vi "AI Config Pane.vi"(6 "_SubPanelMessages":refnum<notifier>, 9 "_myEmbeddedToFrameEvent":T7, 10 "_myEmbedded.Exit":refnum<user-event>, 11 "-Property Bundle":cluster{"Name":string, "Value":variant}[](array[cluster])) -> (1 "_Connection Informations":T1, 2 "_Scripter Input":T9)   [LabVIEW 2021]
uses:
  <vilib>/myRIO/Common/Express VI Framework/xctls/myRIO Channel List/myRIO Channel List.xctl
  <vilib>/myRIO/Common/Express VI Framework/typedefs/Config Pane to Framework Ref.ctl
  <vilib>/myRIO/Common/Express VI Framework/typedefs/Data Validate Ref.ctl
  <vilib>/myRIO/Common/Express VI Framework/typedefs/Scripter Input.ctl
  <vilib>/myRIO/Common/Express VI Framework/typedefs/WireThrough Terminal Names.ctl
  <vilib>/myRIO/Common/Express VI Framework/typedefs/Instrument Driver Method Descriptor Array.ctl
  <vilib>/myRIO/Common/Express VI Framework/typedefs/Instrument Driver Method Descriptor.ctl
  <vilib>/myRIO/Common/Express VI Framework/typedefs/Sub Panel Messages.ctl
  <vilib>/myRIO/Common/Express VI Framework/typedefs/Connection Informations.ctl
  <vilib>/myRIO/Common/Instrument Driver Framework/Utilities/typedefs/Channel Types.ctl
  <vilib>/myRIO/Common/Profile Manager Framework/typedefs/Channel Type Profile.ctl
  <vilib>/myRIO/Common/Profile Manager Framework/typedefs/Channel Info.ctl
panel:
  in  "Range Indexes":i32[](array[numeric])
  in  "Selected Channel List":T2[](xcontrol)=[{"Channel Name"=0, "Channel Alias"="", "Remove Channel"=FALSE, "Index"=0}]
  in  "_Default Alias String":string
  in  "_VI Default Name (Edit and make value default)":string="Analog input (1 sample)"
  in  "Name:":string caption="Node name:"
  in  "_WireThrough Info (Edit and make value default)":T4={"WireThrough Top In"="AI Ref In", "WireThrough Bottom In"="error in (no error)", "WireThrough Top Out"="AI Ref Out", "WireThrough Bottom Out"="error out"}
  in  "_Template Array (Edit and make value default)":T5=[{"Function Name"="Smart Open", "VI Path"=path "<vilib>/myRIO/Instrument Drivers/Onboard IO/AI/vis", "Script"=TRUE, "Inputs"=[{"name"="Channel Names", "value"=variant, "Config Pane Only"=TRUE, "Build Array"=FALSE, "Bundle Cluster"=FALSE, "Show Term"=FALSE, "alias"=[], "Required Input"=FALSE}], "Outputs"=[], "VI Class"=enum."Open", "Controls Refs[]"=[], "Inline"=FALSE}, {"Function Name"="Open", "VI Path"=path "<vilib>/myRIO/Instrument Drivers/Onboard IO/AI/vis", "Script"=FALSE, "Inputs"=[{"name"="Channel Names", "value"=variant, "Config Pane Only"=TRUE, "Build Array"=FALSE, "Bundle Cluster"=FALSE, "Show Term"=FALSE, "alias"=[], "Required Input"=FALSE}], "Outputs"=[], "VI Class"=enum."Open", "Controls Refs[]"=[], "Inline"=FALSE}, {"Function Name"="Read", "VI Path"=path "<vilib>/myRIO/Instrument Drivers/Onboard IO/AI/vis", "Script"=TRUE, "Inputs"=[], "Outputs"=[{"name"="Values", "value"=variant, "Show Term"=TRUE, "Index Array"=TRUE, "Unbundle Cluster"=FALSE, "alias"=[]}], "VI Class"=enum."Data", "Controls Refs[]"=[], "Inline"=FALSE}, {"Function Name"="Close", "VI Path"=path "<vilib>/myRIO/Instrument Drivers/Onboard IO/AI/vis", "Script"=FALSE, "Inputs"=[], "Outputs"=[], "VI Class"=enum."Close", "Controls Refs[]"=[], "Inline"=FALSE}]
  in  "_Test Close":bool
  # "User Visible Area"
  # "NOTE: Tab Order has been set\nfor this Front Panel.\n1. Name: (string control)\n2. Add Channel (button)\n3. Selected Channel List (array)\n\nAll other controls are excluded \nfrom Tabbing order\n\nTo exlude a control from context\nhelp prefix its label text with a '-'"
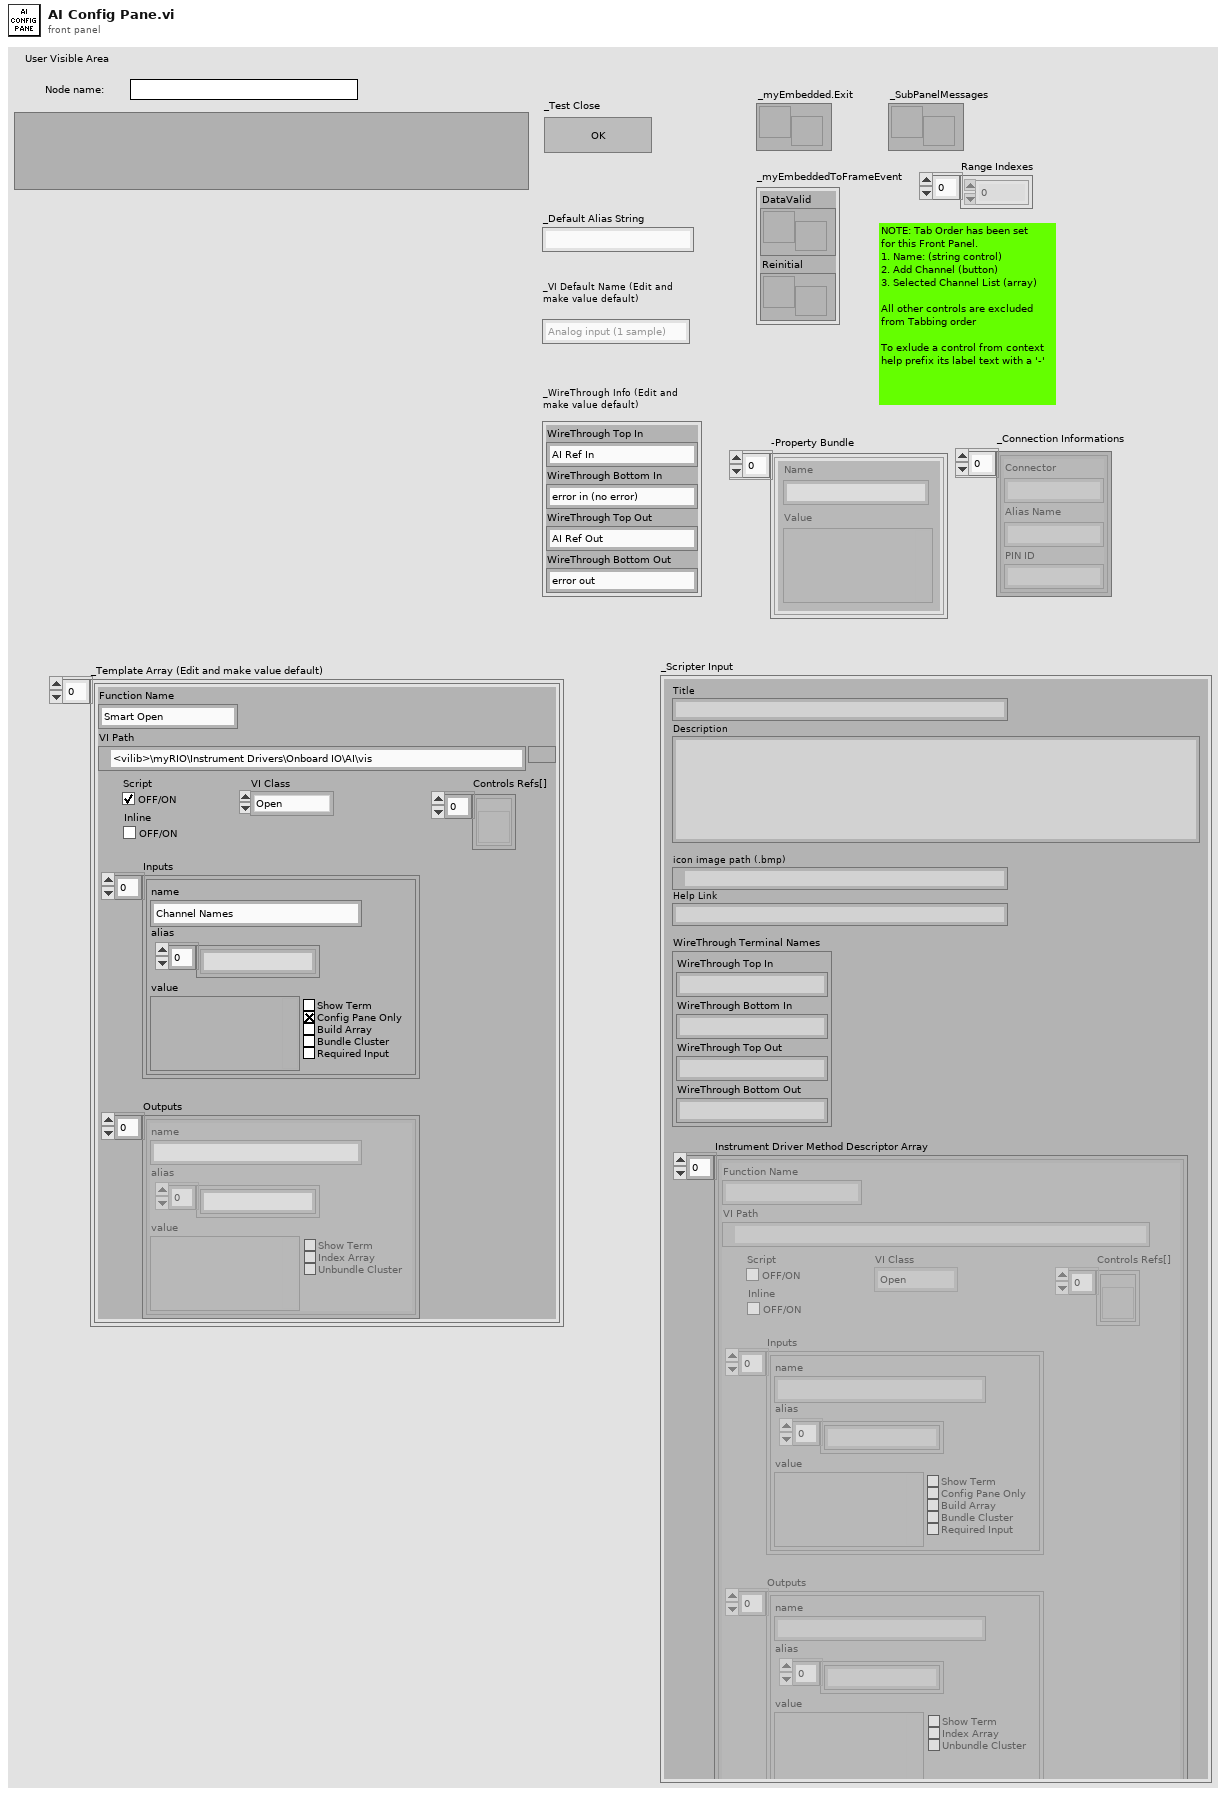
[diagram p1: front panel]
types:
  T1 = typedef "Connection Informations.ctl" = cluster{"Connector":string, "Alias Name":string, "PIN ID":string}[]
  T2 = typedef "myRIO Channel List.xctl/Channel Data.ctl" = cluster{"Channel Name":u16, "Channel Alias":string, "Remove Channel":T3, "Index":i32}
  T3 = typedef "myRIO Channel List.xctl/Remove Channel.ctl" = bool
  T4 = typedef "WireThrough Terminal Names.ctl" = cluster{"WireThrough Top In":string, "WireThrough Bottom In":string, "WireThrough Top Out":string, "WireThrough Bottom Out":string}
  T5 = typedef "Instrument Driver Method Descriptor Array.ctl" = T6[]
  T6 = typedef "Instrument Driver Method Descriptor.ctl" = cluster{"Function Name":string, "VI Path":path, "Script":bool, "Inputs":cluster{"name":string, "value":variant, "Config Pane Only":bool, "Build Array":bool, "Bundle Cluster":bool, "Show Term":bool, "alias":string[], "Required Input":bool}[], "Outputs":cluster{"name":string, "value":variant, "Show Term":bool, "Index Array":bool, "Unbundle Cluster":bool, "alias":string[]}[], "VI Class":enum16{"Open", "Configure", "Data", "Manage", "Close"}, "Controls Refs[]":refnum<vi>[], "Inline":bool}
  T7 = typedef "Config Pane to Framework Ref.ctl" = cluster{"DataValid":T8, "Reinitial":refnum<user-event>}
  T8 = typedef "Data Validate Ref.ctl" = refnum<user-event>
  T9 = typedef "Scripter Input.ctl" = cluster{"Title":string, "Description":string, "icon image path (.bmp)":path, "Help Link":string, "WireThrough Terminal Names":T4, "Instrument Driver Method Descriptor Array":T5}
  T10 = typedef "Channel Types.ctl" = enum32{"Unknown", "AI", "AO", "DIO - DI", "DIO", "DIO - DO", "I2C", "PWM", "Encoder", "SPI", "UART", "Accelerometer", "DIO - LED", "DIO - Button", "AI (N Samples)", "AudioIn (N Samples)", "AO (N Samples)", "AudioOut (N Samples)", "DI (N Samples)", "DO (N Samples)", "AI IRQ", "DI IRQ", "Timer IRQ", "RSL", "Relay", "CAN", "AI (Continuous)", "AO (Continuous)"}
  T11 = typedef "Channel Type Profile.ctl" = cluster{"Channel Type":T10, "No. of Channels":dbl, "Channel List":T12[]}
  T12 = typedef "Channel Info.ctl" = cluster{"Channel Name":string, "Alias":string, "Used?":bool, "Not Support?":bool, "Property Bundle":cluster{"Name":string, "Value":variant}[]}
  T13 = typedef "Sub Panel Messages.ctl" = enum16{"Initialized"}
  T14 = cluster{"name":string, "value":variant, "Config Pane Only":bool, "Build Array":bool, "Bundle Cluster":bool, "Show Term":bool, "alias":string[], "Required Input":bool}
  T15 = cluster{"Connector":string, "Alias Name":string, "PIN ID":string}[]
  T16 = cluster{"name":string, "value":variant, "Config Pane Only":bool, "Build Array":bool, "Bundle Cluster":bool, "Show Term":bool, "alias":string[], "Required Input":bool}[]
  T17 = cluster{"name":string, "value":variant, "Show Term":bool, "Index Array":bool, "Unbundle Cluster":bool, "alias":string[]}[]
  T18 = cluster{"name":string, "value":variant, "Show Term":bool, "Index Array":bool, "Unbundle Cluster":bool, "alias":string[]}
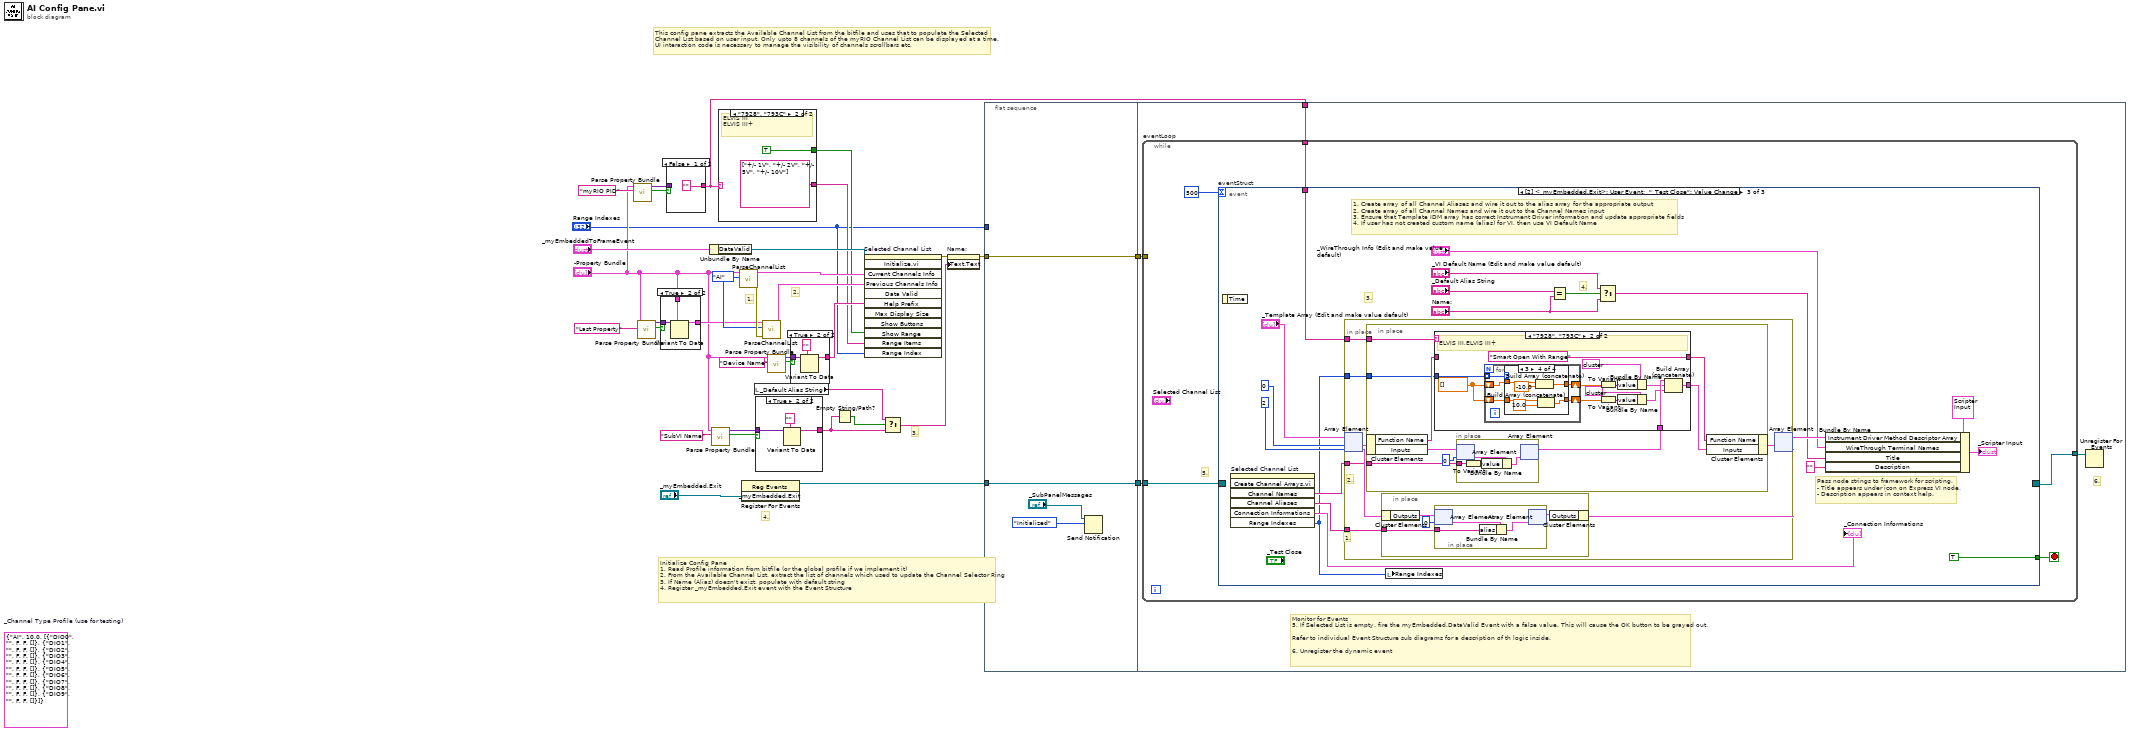
[diagram p0: block diagram]
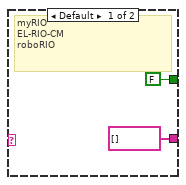
[diagram p2: hidden frame]
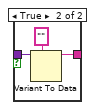
[diagram p3: hidden frame]
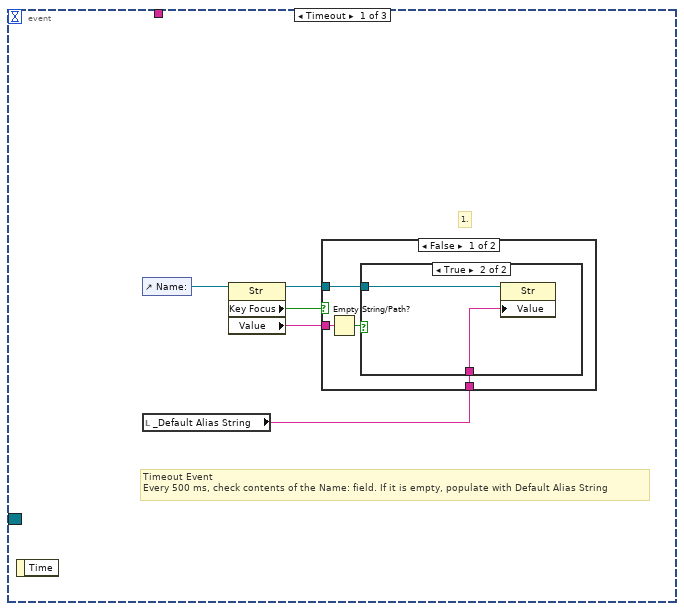
[diagram p4: hidden frame]
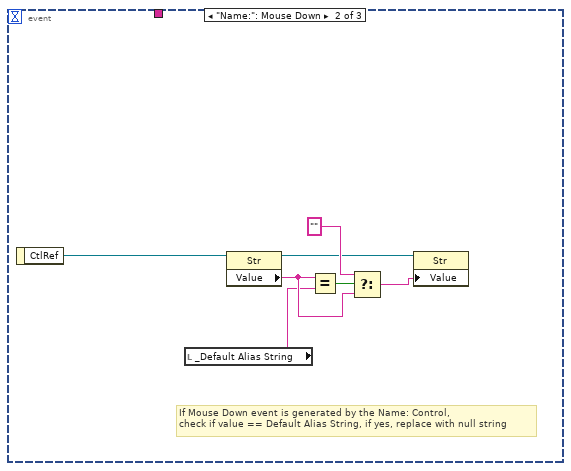
[diagram p7: hidden frame]
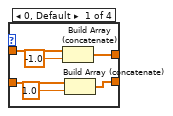
[diagram p9: hidden frame]
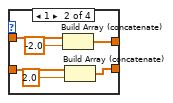
[diagram p10: hidden frame]
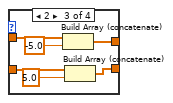
[diagram p11: hidden frame]
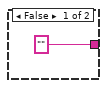
[diagram p14: hidden frame]
diagram:
  w18 = Channel_Types."AI" ("Channel to Read")
  (unwired) T11 {"Channel Type"=enum."AI", "No. of Channels"=10.0, "Channel List"=[{"Channel Name"="DIO0", "Alias"="", "Used?"=FALSE, "Not Support?"=FALSE, "Property Bundle"=[]}, {"Channel Name"="DIO1", "Alias"="", "Used?"=FALSE, "Not Support?"=FALSE, "Property Bundle"=[]}, {"Channel Name"="DIO2", "Alias"="", "Used?"=FALSE, "Not Support?"=FALSE, "Property Bundle"=[]}, {"Channel Name"="DIO3", "Alias"="", "Used?"=FALSE, "Not Support?"=FALSE, "Property Bundle"=[]}, {"Channel Name"="DIO4", "Alias"="", "Used?"=FALSE, "Not Support?"=FALSE, "Property Bundle"=[]}, {"Channel Name"="DIO5", "Alias"="", "Used?"=FALSE, "Not Support?"=FALSE, "Property Bundle"=[]}, {"Channel Name"="DIO6", "Alias"="", "Used?"=FALSE, "Not Support?"=FALSE, "Property Bundle"=[]}, {"Channel Name"="DIO7", "Alias"="", "Used?"=FALSE, "Not Support?"=FALSE, "Property Bundle"=[]}, {"Channel Name"="DIO8", "Alias"="", "Used?"=FALSE, "Not Support?"=FALSE, "Property Bundle"=[]}, {"Channel Name"="DIO9", "Alias"="", "Used?"=FALSE, "Not Support?"=FALSE, "Property Bundle"=[]}]}  # _Channel Type Profile (use for testing)
  # "3."
  # "2."
  # "1."
  # "This config pane extracts the Available Channel List from the bitfile and uses that to populate the Selected \nChannel List based on user input. Only upto 8 channels of the myRIO Channel List can be displayed at a time. \nUI interaction code is necessary to manage the visibility of channels scrollbars etc."
  # "4."
  # "Initialize Config Pane\n1. Read Profile information from bitfile (or the global profile if we implement it)\n2. From the Available Channel List, extract the list of channels which used to update the Channel Selector Ring\n3. If Name (Alias) doesn't exist, populate with default string\n4. Register _myEmbedded.Exit event with the Event Structure"
  n1 = call <vilib>:"Parse Property Bundle.vi"("Name"="myRIO PID", "Property Bundle"="-Property Bundle") -> ("Found?"=w1:bool, "Value"=w7:variant)  [unwired: 8 in]
  n2 = call <vilib>:"Parse Property Bundle.vi"("Name"="Last Property", "Property Bundle"="-Property Bundle") -> ("Found?"=w20:bool, "Value"=w21:variant)  [unwired: 8 in]
  n3 = case shown="True" w20 {
    tunnel: w21 -> [_ w38]
    tunnel: [_ w37] -> w17
    tunnel: "-Property Bundle" -> [_ w36]
    frame False {
    }
    frame True {
      n4 = Variant To Data(type=w36, Variant=w38) -> (data=w37:cluster{"Name":string, "Value":variant}[])  [unwired: 1 in, 1 out]
    }
  }
  n5 = case shown="False" w1 {
    tunnel: w7 -> [_ w42]
    tunnel: ["" ("Name") w41] -> w2
    frame False {
    }
    frame True {
      n6 = Variant To Data(type="" ("Name"), Variant=w42) -> (data=w41:string)  [unwired: 1 in, 1 out]
    }
  }
  n7 = Unbundle By Name("_myEmbeddedToFrameEvent") -> ("DataValid"=w11:T8)
  n8 = call <vilib>:"Parse Property Bundle.vi"("Name"="SubVI Name", "Property Bundle"="-Property Bundle") -> ("Found?"=w29:bool, "Value"=w30:variant)  [unwired: 8 in]
  n9 = case shown="\"7928\", \"793C\"" w2 {
    tunnel: [FALSE TRUE] -> w4
    tunnel: [string[] [] ("Range Items") string[] ["+/- 1V", "+/- 2V", "+/- 5V", "+/- 10V"] ("Range Items")] -> w5
    frame Default {
      # "myRIO\nEL-RIO-CM\nroboRIO"
    }
    frame "7928", "793C" {
      # "ELVIS III\nELVIS III+"
    }
  }
  n10 = call <vilib>:"ParseChannelList.vi"("Channel to Read"=w18, "_Property Bundle"="-Property Bundle") -> ("error out"=w19:errorcluster, "Channel List Out"=w23:T12[])  [unwired: 7 in, 1 out]
  n11 = register-events("_myEmbedded.Exit") -> (reference out=w27:refnum<event-registration>)  [unwired: 2 in, 1 out]
  n12 = local read "_Default Alias String"() -> (w25:string)
  n13 = case shown="True" w29 {
    tunnel: w30 -> [_ w50]
    tunnel: ["" ("Name") w48] -> w28
    frame False {
    }
    frame True {
      n14 = Variant To Data(type="" ("Name"), Variant=w50) -> (data=w48:string)  [unwired: 1 in, 1 out]
    }
  }
  n15 = call <vilib>:"ParseChannelList.vi"("error in (no error)"=w19, "Channel to Read"=w18, "_Property Bundle"=w17) -> ("Channel List Out"=w16:T12[])  [unwired: 6 in, 2 out]
  n16 = call <vilib>:"Parse Property Bundle.vi"("Name"="Device Name", "Property Bundle"="-Property Bundle") -> ("Found?"=w15:bool, "Value"=w14:variant)  [unwired: 8 in]
  n17 = case shown="True" w15 {
    tunnel: w14 -> [_ w53]
    tunnel: [_ w52] -> w12
    frame False {
    }
    frame True {
      n18 = Variant To Data(type="", Variant=w53) -> (data=w52:string)  [unwired: 1 in, 1 out]
    }
  }
  n19 = Empty String/Path?(string/path=w28) -> (empty?=w34:bool)
  n20 = invoke on="Selected Channel List" class="myRIO Channel List (strict)" method="Initialize.vi"("Current Channels Info"=w23, "Previous Channels Info"=w16, "Data Valid"=w11, "Help Prefix"=w12, "Show Range"=w4, "Range Items"=w5, "Range Index"="Range Indexes") -> (error out=w26:errorcluster)  [unwired: 5 in, 11 out]
  n21 = Select(t=w25, s=w34, f=w28) -> (s? t:f=w33:string)
  n22 = property on="Name:" class="Str"(error in=w26, "Text.Text"=w33) -> (error out=w32:errorcluster)  [unwired: 1 in, 1 out]
  n23 = flat-sequence {
    tunnel: w27 -> [w56]
    tunnel: w32 -> [w57]
    tunnel: [w57] -> w10
    tunnel: [w56] -> w9
    tunnel: "Range Indexes" -> [_]
    tunnel: w10 -> [w60]
    tunnel: w9 -> [w59]
    tunnel: w2 -> [w58]
    frame #0 {
      n24 = Send Notification(notification=Sub_Panel_Messages."Initialized", notifier="_SubPanelMessages") -> ()  [unwired: 1 in, 2 out]
    }
    frame #1 {
      # "Monitor for Events\n5. If Selected List is empty, fire the myEmbedded.DataValid Event with a false value. This will cause the OK button to be grayed out.\n\nRefer to individual Event Structure sub diagrams for a description of th logic inside.\n\n6. Unregister the dynamic event"
      # "6."
      n25 = while "eventLoop" {
        tunnel: w59 -> [w65]
        tunnel: [w64] -> w61
        tunnel: w60 -> [_]
        tunnel: w58 -> [w62]
        stop <- w66 stop-if-true
        # "5."
        n26 = event "eventStruct" shown="[2] <_myEmbedded.Exit>: User Event;  \"_Test Close\": Value Change" {
          selector: w65 -> [_ _ _]
          dyn-events: [_ _ _] -> w64
          timeout: 500 -> [_ _ _]
          tunnel: [_ _ TRUE ("_Test Close")] -> w66
          tunnel: w62 -> [_ _ w86]
          event Timeout {
            # "Timeout Event\nEvery 500 ms, check contents of the Name: field. If it is empty, populate with Default Alias String"
            # "1."
            n27 = event-data() -> ()  [unwired: 1 in, 1 out]
            n28 = control-ref of="Name:"() -> (w69:refnum<vi>)
            n29 = local read "_Default Alias String"() -> (w67:string)
            n30 = property on="Property Node" class="Str"(reference=w69) -> (reference out=w68:refnum<vi>, "Key Focus"=w70:bool, "Value"=w71:string)  [unwired: 1 in, 1 out]
            n31 = case shown="False" w70 {
              tunnel: w71 -> [w75 _]
              tunnel: w68 -> [w73 _]
              tunnel: w67 -> [w72 _]
              frame False {
                n32 = Empty String/Path?(string/path=w75) -> (empty?=w74:bool)
                n33 = case shown="True" w74 {
                  tunnel: w73 -> [_ w77]
                  tunnel: w72 -> [_ w76]
                  frame False {
                  }
                  frame True {
                    n34 = property on="Property Node" class="Str"(reference=w77, "Value"=w76) -> ()  [unwired: 1 in, 2 out]
                  }
                }
              }
              frame True {
              }
            }
          }
          event "Name:": Mouse Down {
            # "If Mouse Down event is generated by the Name: Control,\ncheck if value == Default Alias String, if yes, replace with null string"
            n35 = event-data() -> ("CtlRef"=w84:refnum<vi>)  [unwired: 1 in]
            n36 = local read "_Default Alias String"() -> (w78:string)
            n37 = property class="Str"(reference=w84) -> (reference out=w80:refnum<vi>, "Value"=w79:string)  [unwired: 1 in, 1 out]
            n38 = Equal?(x=w79, y=w78) -> (x = y?=w83:bool)
            n39 = Select(t="", s=w83, f=w79) -> (s? t:f=w81:string)
            n40 = property class="Str"(reference=w80, "Value"=w81) -> ()  [unwired: 1 in, 2 out]
          }
          event User Event; "_Test Close": Value Change {
            # "2."
            # "1."
            # "1. Create array of all Channel Aliases and wire it out to the alias array for the appropriate output\n2. Create array of all Channel Names and wire it out to the Channel Names input\n3. Ensure that Template IDM array has correct Instrument Driver information and update appropriate fields\n4. If user has not created custom name (alias) for VI, then use VI Default Name"
            # "4."
            # "3."
            # "Pass node strings to framework for scripting.\n- Title appears under icon on Express VI node.\n- Description appears in context help."
            n41 = event-data() -> ()  [unwired: 1 in, 1 out]
            n42 = invoke on="Selected Channel List" class="myRIO Channel List (strict)" method="Create Channel Arrays.vi"() -> ("Channel Names"=w89:string[], "Channel Aliases"=w88:string[], "Connection Informations"=→"_Connection Informations":T15, "Range Indexes"=w85:i32[])  [unwired: 7 in, 3 out]
            n43 = in-place {
              in-place-border: w89 -> [w107]
              in-place-border: w88 -> [w106]
              in-place-border: w86 -> [w105]
              in-place-border: w85 -> [w104]
              n44 = in-place-array #1("_Template Array (Edit and make value default)", 0, 2) -> (w111:T6, w109:T6)
              n45 = in-place {
                in-place-border: w107 -> [w126]
                in-place-border: w105 -> [w124]
                in-place-border: w104 -> [w120]
                n46 = in-place-cluster #2(w111) -> ("Function Name"=w123:string, "Inputs"=w127:T16)
                n47 = in-place {
                  in-place-border: w126 -> [w172]
                  n48 = in-place-array #3(w127, 0) -> (w175:T14)
                  n49 = To Variant(anything=w172) -> (Variant=w173:variant)
                  n50 = Bundle By Name(cluster=w175, "value"=w173) -> (w174:T14)
                  n51 = in-place-array #3(w174) -> (w121:T16)  [unwired: 1 out]
                }
                n52 = case shown="\"7928\", \"793C\"" w124 {
                  tunnel: w123 -> [w129 _]
                  tunnel: [w129 "Smart Open With Range"] -> w122
                  tunnel: w121 -> [w128 w141]
                  tunnel: w120 -> [_ w140]
                  tunnel: [w128 w130] -> w119
                  frame Default {
                    # "myRIO,EL-RIO-CM,roboRIO"
                  }
                  frame "7928", "793C" {
                    w139 = dbl[] []
                    # "ELVIS III,ELVIS III+"
                    n53 = for {
                      tunnel: w140 -> [w147] mode=indexing
                      shift-right: [w145] -> w137
                      shift-left: w139 -> [w146]
                      shift-right: [w143] -> w134
                      shift-left: w139 -> [w144]
                      n54 = case shown="3" w147 {
                        tunnel: w146 -> [w151 w157 w163 w169]
                        tunnel: [w150 w156 w162 w168] -> w145
                        tunnel: w144 -> [w149 w155 w161 w167]
                        tunnel: [w148 w154 w160 w166] -> w143
                        frame 0, Default {
                          n55 = Build Array (concatenate)(w151, -1.0) -> (w150:dbl[])
                          n56 = Build Array (concatenate)(w149, 1.0) -> (w148:dbl[])
                        }
                        frame 1 {
                          n57 = Build Array (concatenate)(w157, -2.0) -> (w156:dbl[])
                          n58 = Build Array (concatenate)(w155, 2.0) -> (w154:dbl[])
                        }
                        frame 2 {
                          n59 = Build Array (concatenate)(w163, -5.0) -> (w162:dbl[])
                          n60 = Build Array (concatenate)(w161, 5.0) -> (w160:dbl[])
                        }
                        frame 3 {
                          n61 = Build Array (concatenate)(w169, -10.0) -> (w168:dbl[])
                          n62 = Build Array (concatenate)(w167, 10.0) -> (w166:dbl[])
                        }
                      }
                    }
                    n63 = To Variant(anything=w137) -> (Variant=w138:variant)
                    n64 = To Variant(anything=w134) -> (Variant=w135:variant)
                    n65 = Bundle By Name(cluster=T14 {"name"="Min Value", "value"=variant, "Config Pane Only"=TRUE, "Build Array"=FALSE, "Bundle Cluster"=FALSE, "Show Term"=FALSE, "alias"=[], "Required Input"=FALSE} ("element"), "value"=w138) -> (w132:T14)
                    n66 = Bundle By Name(cluster=T14 {"name"="Max Value", "value"=variant, "Config Pane Only"=TRUE, "Build Array"=FALSE, "Bundle Cluster"=FALSE, "Show Term"=FALSE, "alias"=[], "Required Input"=FALSE} ("element"), "value"=w135) -> (w131:T14)
                    n67 = Build Array (concatenate)(w141, w132, w131) -> (w130:T16)
                  }
                }
                n68 = in-place-cluster #2("Function Name"=w122, "Inputs"=w119) -> (w110:T6)
              }
              n69 = in-place {
                in-place-border: w106 -> [w114]
                n70 = in-place-cluster #4(w109) -> ("Outputs"=w115:T17)
                n71 = in-place {
                  in-place-border: w114 -> [w116]
                  n72 = in-place-array #5(w115, 0) -> (w118:T18)
                  n73 = Bundle By Name(cluster=w118, "alias"=w116) -> (w117:T18)
                  n74 = in-place-array #5(w117) -> (w113:T17)  [unwired: 1 out]
                }
                n75 = in-place-cluster #4("Outputs"=w113) -> (w108:T6)
              }
              n76 = in-place-array #1(w110, w108) -> (w101:T5)  [unwired: 2 out]
            }
            n77 = local write "Range Indexes"(w85) -> ()
            n78 = Equal?(x="_Default Alias String", y="Name:") -> (x = y?=w93:bool)
            n79 = Select(t="_VI Default Name (Edit and make value default)", s=w93, f="Name:") -> (s? t:f=w91:string)
            n80 = Bundle By Name(cluster=T9 {"Title"="", "Description"="", "icon image path (.bmp)"=path "", "Help Link"="", "WireThrough Terminal Names"={"WireThrough Top In"="", "WireThrough Bottom In"="", "WireThrough Top Out"="", "WireThrough Bottom Out"=""}, "Instrument Driver Method Descriptor Array"=[]} ("Scripter Input"), "Instrument Driver Method Descriptor Array"=w101, "WireThrough Terminal Names"="_WireThrough Info (Edit and make value default)", "Title"=w91, "Description"="" ("Title")) -> (→"_Scripter Input":T9)
          }
        }
      }
      n81 = Unregister For Events(event registration refnum=w61) -> ()  [unwired: 1 in, 1 out]
    }
  }
